vi "4.vi"() -> ()   [LabVIEW 2017]
panel:
  out "Gauge":dbl(knob) scale=0.0..255.0
  out "Thermometer":dbl(slide) scale=0.0..255.0
  out "Numeric":dbl
  in  "Array":bool[](array[boolean])
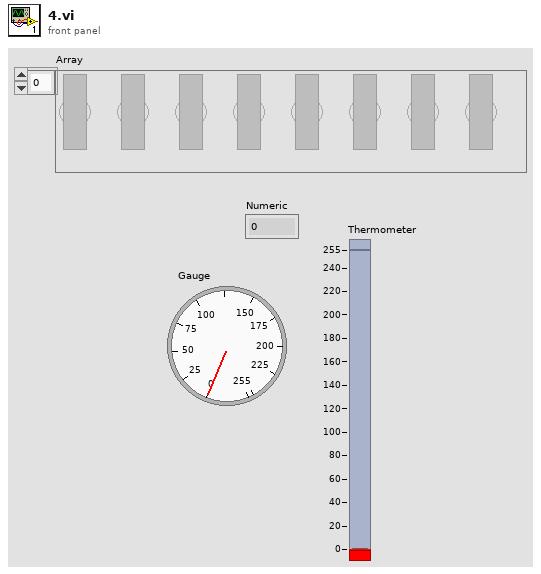
[diagram p1: front panel]
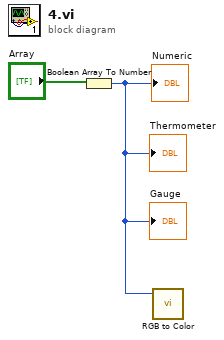
[diagram p0: block diagram]
diagram:
  n1 = Boolean Array To Number(Boolean array="Array") -> (number=w1:u32)
  "Numeric" <- w1
  "Thermometer" <- w1
  "Gauge" <- w1
  n2 = call <vilib>:"RGB to Color.vi"("R"=w1) -> ()  [unwired: 2 in, 1 out]
